vi "test-linear-filter-ALL.vi"(8 "error in (no error)":errorcluster) -> (0 "error out":errorcluster, 3 "ALL TESTS GOOD":bool)   [LabVIEW 2019]
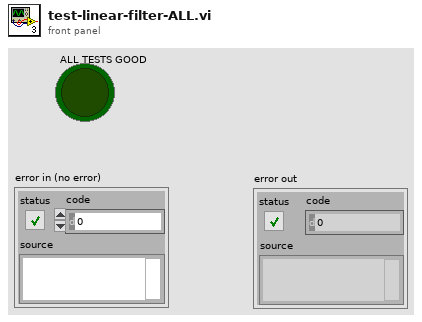
[diagram p1: front panel]
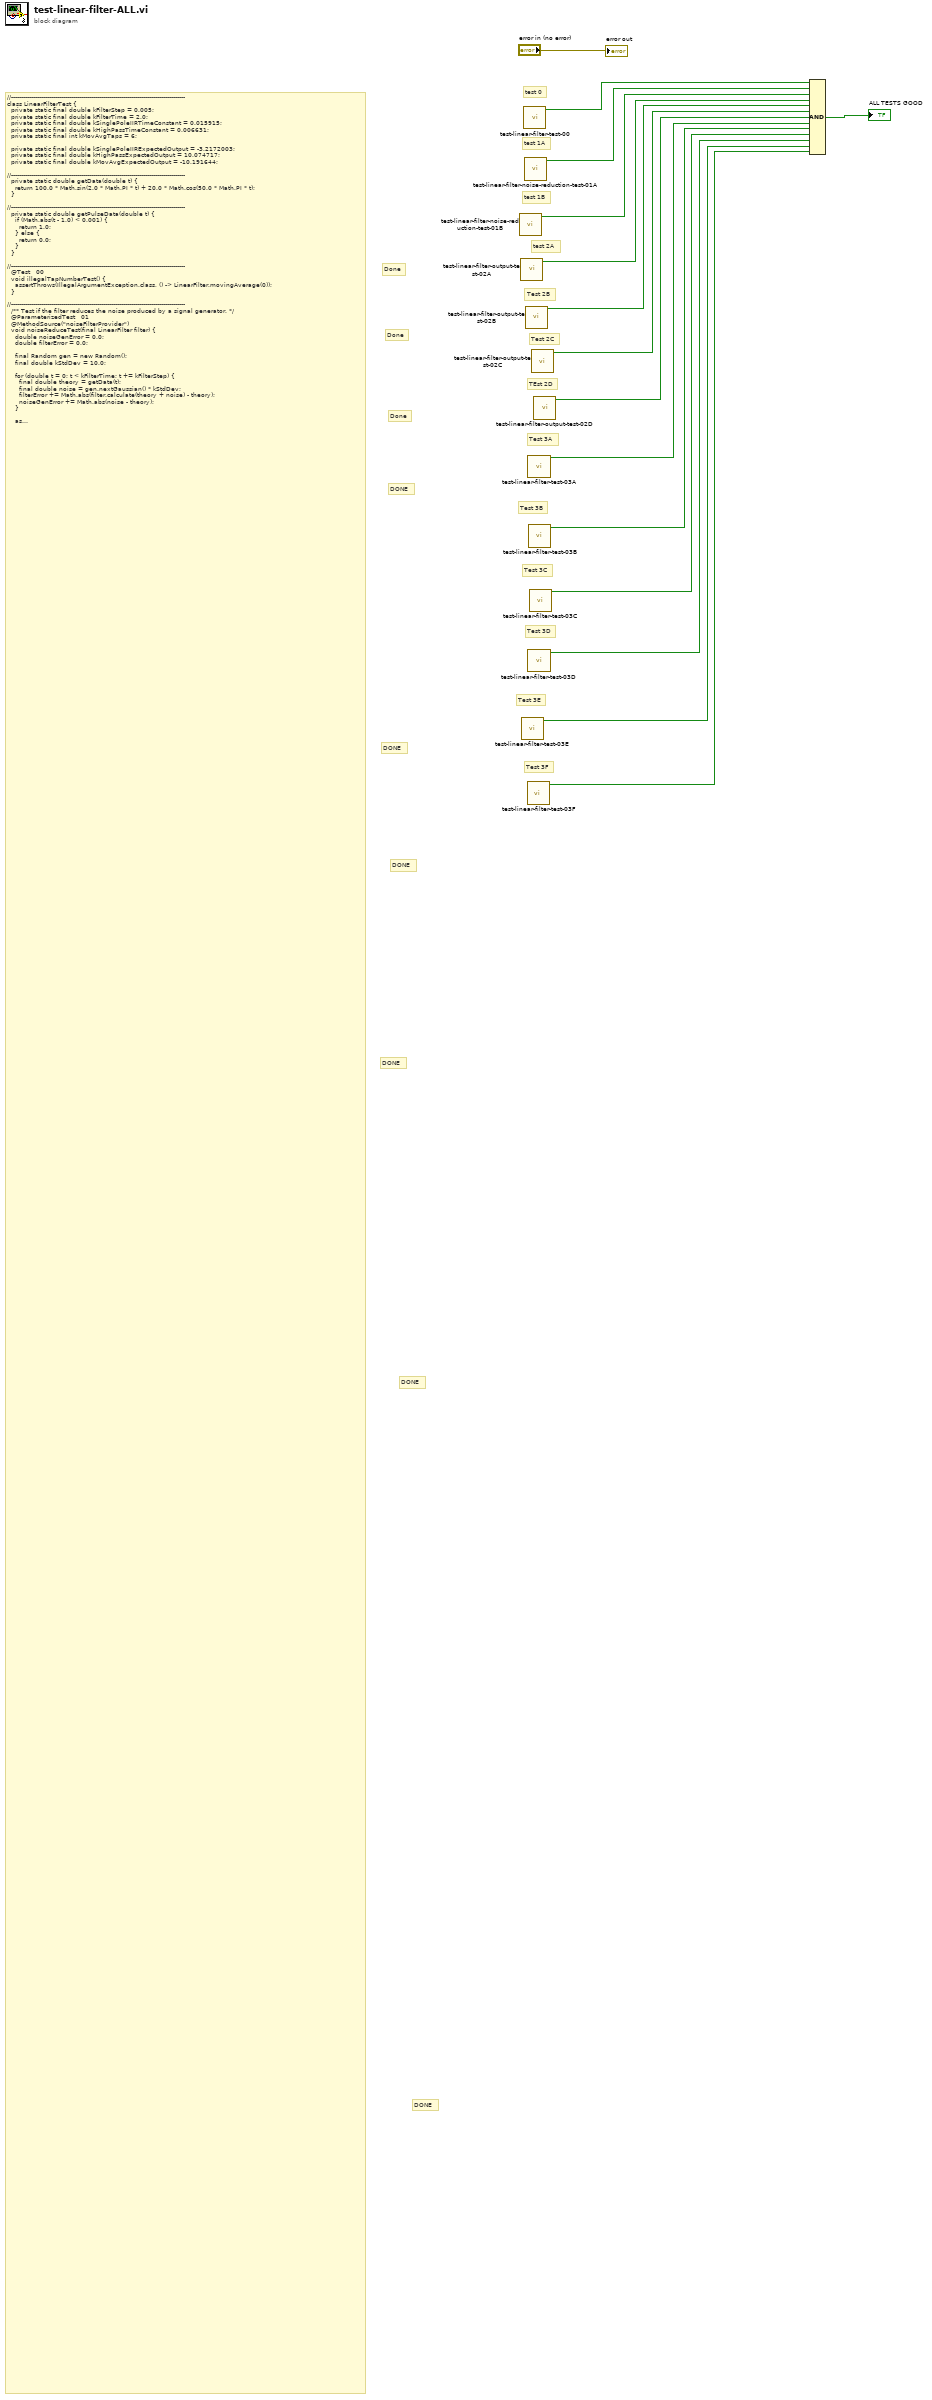
[diagram p0: block diagram]
diagram:
  # "Test 3F"
  # "Test 3E"
  # "Test 3D"
  # "Test 3C"
  # "Test 3B"
  # "Test 3A"
  # "DONE"
  # "DONE"
  # "DONE"
  # "TEst 2D"
  # "Test 2C"
  # "Test 2B"
  # "test 2A"
  # "DONE"
  # "DONE"
  # "test 1B"
  # "test 1A"
  # "DONE"
  # "Done"
  # "Done"
  # "Done"
  # "test 0"
  # "//---------------------------------------------------------------------------------------\nclass LinearFilterTest {\n  private static final double kFilterStep = 0.005;\n  private static final double kFilterTime = 2.0;\n  private static final double kSinglePoleIIRTimeConstant = 0.015915;\n  private static final double kHighPassTimeConstant = 0.006631;\n  private static final int kMovAvgTaps = 6;\n\n  private static final double kSinglePoleIIRExpectedOutput = -3.2172003;\n  private static final double kHighPassExpectedOutput = 10.074717;\n  private static final double kMovAvgExpectedOutput = -10.191644;\n\n//---------------------------------------------------------------------------------------\n  private static double getData(double t) {\n    return 100.0 * Math.sin(2.0 * Math.PI * t) + 20.0 * Math.cos(50.0 * Math.PI * t);\n  }\n\n//---------------------------------------------------------------------------------------\n  private static double getPulseData(double t) {\n    if (Math.abs(t - 1.0) < 0.001) {\n      return 1.0;\n    } else {\n      return 0.0;\n    }\n  }\n\n//---------------------------------------------------------------------------------------\n  @Test   00\n  void illegalTapNumberTest() {\n    assertThrows(IllegalArgumentException.class, () -> LinearFilter.movingAverage(0));\n  }\n\n//---------------------------------------------------------------------------------------\n  /** Test if the filter reduces the noise produced by a signal generator. */\n  @ParameterizedTest   01\n  @MethodSource(\"noiseFilterProvider\")\n  void noiseReduceTest(final LinearFilter filter) {\n    double noiseGenError = 0.0;\n    double filterError = 0.0;\n\n    final Random gen = new Random();\n    final double kStdDev = 10.0;\n\n    for (double t = 0; t < kFilterTime; t += kFilterStep) {\n      final double theory = getData(t);\n      final double noise = gen.nextGaussian() * kStdDev;\n      filterError += Math.abs(filter.calculate(theory + noise) - theory);\n      noiseGenError += Math.abs(noise - theory);\n    }\n\n    assertTrue(\n        noiseGenError > filterError,\n        \"Filter should have reduced noise accumulation from \"\n            + noiseGenError\n            + \" but failed. The filter error was \"\n            + filterError);\n  }\n\n//---------------------------------------------------------------------------------------\n  static Stream<LinearFilter> noiseFilterProvider() {\n    return Stream.of(\n        LinearFilter.singlePoleIIR(kSinglePoleIIRTimeConstant, kFilterStep),\n        LinearFilter.movingAverage(kMovAvgTaps));\n  }\n\n//---------------------------------------------------------------------------------------\n  /** Test if the linear filters produce consistent output for a given data set. */\n  @ParameterizedTest\n  @MethodSource(\"outputFilterProvider\")\n  void outputTest(\n      final LinearFilter filter, final DoubleFunction<Double> data, final double expectedOutput) {\n    double filterOutput = 0.0;\n    for (double t = 0.0; t < kFilterTime; t += kFilterStep) {\n      filterOutput = filter.calculate(data.apply(t));\n    }\n\n    assertEquals(expectedOutput, filterOutput, 5e-5, \"Filter output was incorrect.\");\n  }\n\n//---------------------------------------------------------------------------------------\n  static Stream<Arguments> outputFilterProvider() {\n    return Stream.of(\n        arguments(\n            LinearFilter.singlePoleIIR(kSinglePoleIIRTimeConstant, kFilterStep),\n            (DoubleFunction<Double>) LinearFilterTest::getData,\n            kSinglePoleIIRExpectedOutput),\n        arguments(\n            LinearFilter.highPass(kHighPassTimeConstant, kFilterStep),\n            (DoubleFunction<Double>) LinearFilterTest::getData,\n            kHighPassExpectedOutput),\n        arguments(\n            LinearFilter.movingAverage(kMovAvgTaps),\n            (DoubleFunction<Double>) LinearFilterTest::getData,\n            kMovAvgExpectedOutput),\n        arguments(\n            LinearFilter.movingAverage(kMovAvgTaps),\n            (DoubleFunction<Double>) LinearFilterTest::getPulseData,\n            0.0));\n  }\n\n//---------------------------------------------------------------------------------------\n  /** Test backward finite difference. */\n  @Test  03\n  void backwardFiniteDifferenceTest() {\n    double h = 0.005;\n\n    assertResults(\n        1,\n        2,\n        // f(x) = x²\n        (double x) -> x * x,\n        // df/dx = 2x\n        (double x) -> 2.0 * x,\n        h,\n        -20.0,\n        20.0);\n\n    assertResults(\n        1,\n        2,\n        // f(x) = sin(x)\n        (double x) -> Math.sin(x),\n        // df/dx = cos(x)\n        (double x) -> Math.cos(x),\n        h,\n        -20.0,\n        20.0);\n\n    assertResults(\n        1,\n        2,\n        // f(x) = ln(x)\n        (double x) -> Math.log(x),\n        // df/dx = 1 / x\n        (double x) -> 1.0 / x,\n        h,\n        1.0,\n        20.0);\n\n    assertResults(\n        2,\n        4,\n        // f(x) = x²\n        (double x) -> x * x,\n        // d²f/dx² = 2\n        (double x) -> 2.0,\n        h,\n        -20.0,\n        20.0);\n\n    assertResults(\n        2,\n        4,\n        // f(x) = sin(x)\n        (double x) -> Math.sin(x),\n        // d²f/dx² = -sin(x)\n        (double x) -> -Math.sin(x),\n        h,\n        -20.0,\n        20.0);\n\n    assertResults(\n        2,\n        4,\n        // f(x) = ln(x)\n        (double x) -> Math.log(x),\n        // d²f/dx² = -1 / x²\n        (double x) -> -1.0 / (x * x),\n        h,\n        1.0,\n        20.0);\n  }\n\n//---------------------------------------------------------------------------------------\n  /**\n   * Helper for checking results of backward finite difference.\n   *\n   * @param derivative The order of the derivative.\n   * @param samples The number of sample points.\n   * @param f Function of which to take derivative.\n   * @param dfdx Derivative of f.\n   * @param h Sample period in seconds.\n   * @param min Minimum of f's domain to test.\n   * @param max Maximum of f's domain to test.\n   */\n  void assertResults(\n      int derivative,\n      int samples,\n      DoubleFunction<Double> f,\n      DoubleFunction<Double> dfdx,\n      double h,\n      double min,\n      double max) {\n    var filter = LinearFilter.backwardFiniteDifference(derivative, samples, h);\n\n    for (int i = (int) (min / h); i < (int) (max / h); ++i) {\n      // Let filter initialize\n      if (i < (int) (min / h) + samples) {\n        filter.calculate(f.apply(i * h));\n        continue;\n      }\n\n      // The order of accuracy is O(h^(N - d)) where N is number of stencil\n      // points and d is order of derivative\n      assertEquals(\n          dfdx.apply(i * h),\n          filter.calculate(f.apply(i * h)),\n          10.0 * Math.pow(h, samples - derivative));\n    }\n  }\n}"
  n1 = call "test-linear-filter-noise-reduction-test-01B.vi"() -> ("Passed"=w11:bool)  [unwired: 11 in]
  n2 = call "test-linear-filter-output-test-02A.vi"() -> ("Passed"=w10:bool)  [unwired: 11 in]
  n3 = call "test-linear-filter-test-03E.vi"() -> ("Passed"=w2:bool)  [unwired: 11 in]
  n4 = call "test-linear-filter-test-00.vi"() -> ("Passed"=w13:bool)  [unwired: 11 in]
  n5 = call "test-linear-filter-noise-reduction-test-01A.vi"() -> ("Passed"=w12:bool)  [unwired: 11 in]
  n6 = call "test-linear-filter-output-test-02B.vi"() -> ("Passed"=w9:bool)  [unwired: 11 in]
  n7 = call "test-linear-filter-test-03F.vi"() -> ("Passed"=w1:bool)  [unwired: 11 in]
  n8 = call "test-linear-filter-test-03A.vi"() -> ("Passed"=w6:bool)  [unwired: 11 in]
  n9 = call "test-linear-filter-test-03D.vi"() -> ("Passed"=w3:bool)  [unwired: 11 in]
  n10 = call "test-linear-filter-test-03B.vi"() -> ("Passed"=w5:bool)  [unwired: 11 in]
  n11 = call "test-linear-filter-test-03C.vi"() -> ("Passed"=w4:bool)  [unwired: 11 in]
  n12 = call "test-linear-filter-output-test-02C.vi"() -> ("Passed"=w8:bool)  [unwired: 11 in]
  n13 = call "test-linear-filter-output-test-02D.vi"() -> ("Passed"=w7:bool)  [unwired: 11 in]
  n14 = Compound Arithmetic op=AND(w13, w12, w11, w10, w9, w8, w7, w6, w5, w4, w3, w2, w1) -> (→"ALL TESTS GOOD":bool)
  "error out" <- "error in (no error)"
